vi "Process.vi"(8 "error in (no error)":errorcluster, 11 "SMO.UI":refnum<class "SMO.UI.lvclass">) -> (0 "error out":errorcluster, 3 "SMO.UI out":refnum<class "SMO.UI.lvclass">)   [LabVIEW 2019, in "SMO.UI.lvclass"]
doc: "JKI State Machine Objects (SMO) 1.3.0.56\nJKI - JKI\nCopyright (c) 2017, JKI"
uses:
  SMO.UI.lvclass
  C:/Users/Patrick/Documents/GitHub/Test (LV2019)/lv-venv/lv.lib/vi.lib/JKI/JKI SMO/SMO/SMO.lvclass
  SMO/Typedefs/Parent Call--Enum.ctl
  SMO/SMO.lvclass
  Typedefs/SMO.UI State--enum.ctl
panel:
  in  "self terminate":bool
  out "Copyright":string="JKI State Machine Objects™\nhttp://jki.net/state-machine-objects/\nCopyright (C) 2005-2015, JKI <info@jki.net>\nALL RIGHTS RESERVED\n\nFor instructions on how to use the JKI State Machine Objects, examples and video tutorials, visit:\nhttp://jki.net/state-machine-objects/\n"
  # "JKI SMO UI"
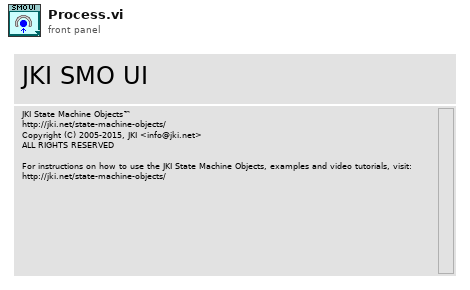
[diagram p1: front panel]
types:
  T1 = typedef "SMO.lvclass/Parent Call--Enum.ctl" = enum16{"Allows parent to run", "Does not request parent to run"}
  T2 = enum32{"invalid app kind", "Development System", "Run Time System", "Student Edition", "Embedded LabVIEW", "Evaluation", "Custom"}
  T3 = enum32{"Invalid", "Standard", "Closed", "Hidden", "Minimized", "Maximized"}
  T4 = typedef "SMO.UI.lvclass/SMO.UI State--enum.ctl" = enum16{"unknown", "Opened", "Closed"}
  T5 = cluster{"Core":cluster{"Current VI Reference":refnum<vi>, "Close Panel on Exit?":bool, "error":errorcluster}, "Self Ref":refnum<class "SMO.UI.lvclass">}
  T6 = cluster{"Current VI Reference":refnum<vi>, "Close Panel on Exit?":bool, "error":errorcluster}
  T7 = typedef "SMO.lvclass/Protected Events.ctl" = cluster{"StopProcesses":refnum<user-event>, "AbortProcesses":refnum<user-event>, "Config Changed":refnum<user-event>, "Dependency":refnum<user-event>}
  T8 = typedef "SMO.UI.lvclass/PrivateEvents--Cluster.ctl" = cluster{"Show-Hide UI":refnum<user-event>}
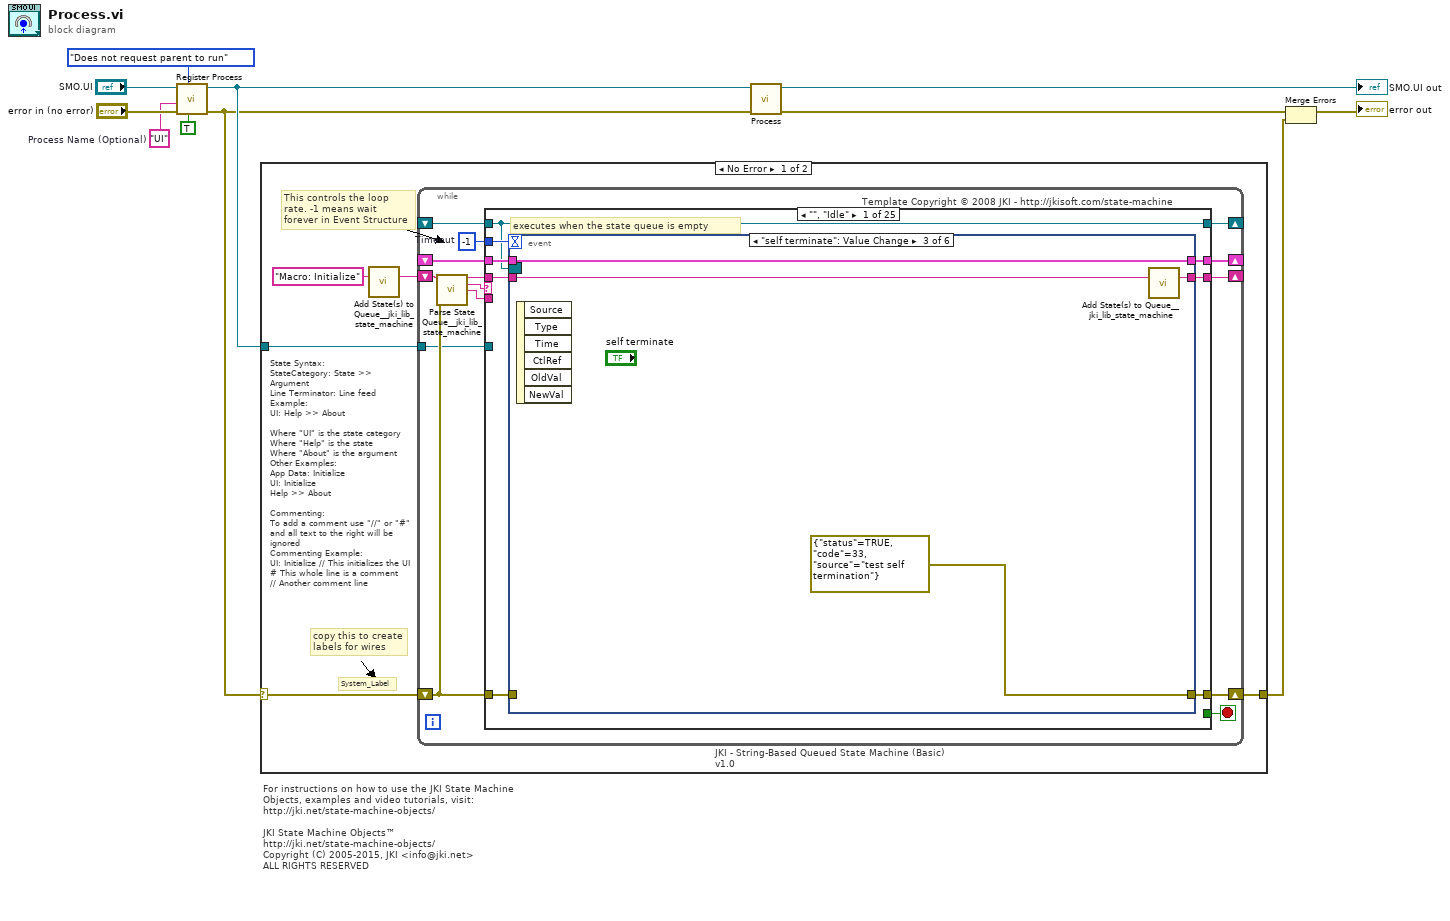
[diagram p0: block diagram]
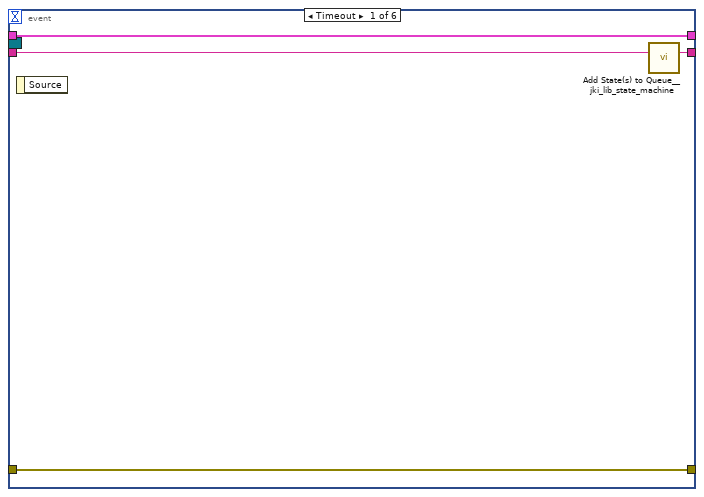
[diagram p2: hidden frame]
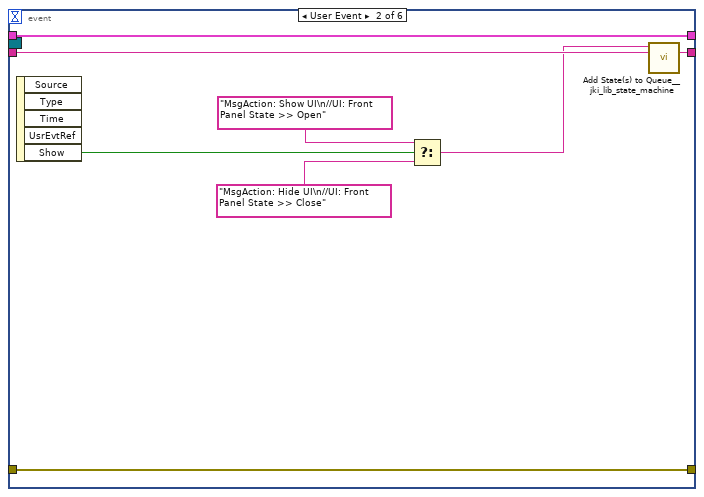
[diagram p3: hidden frame]
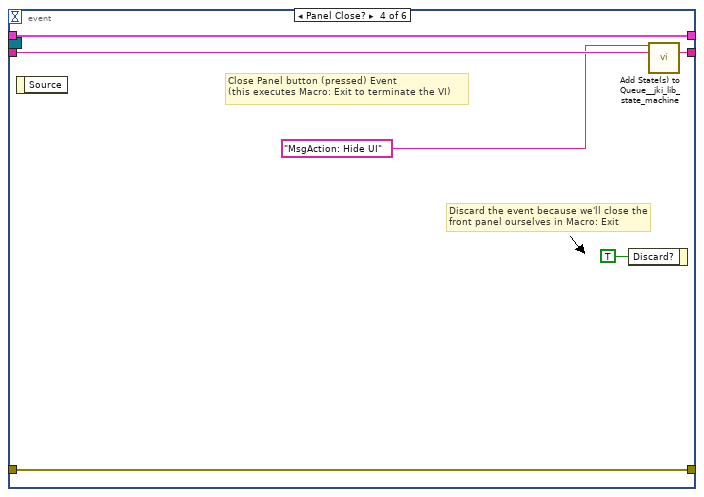
[diagram p4: hidden frame]
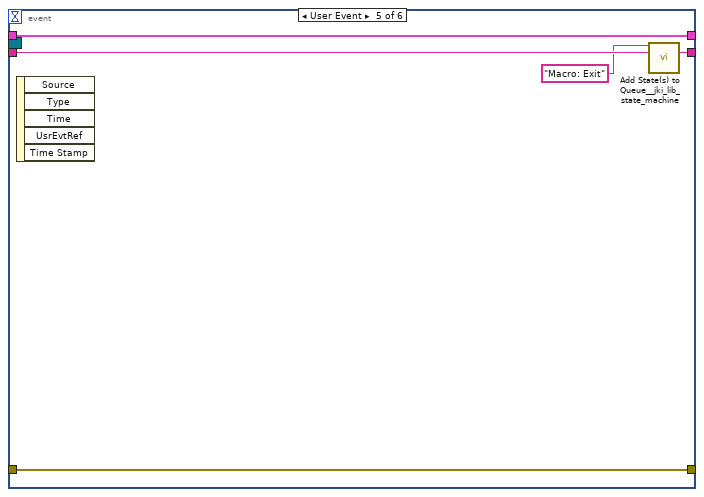
[diagram p5: hidden frame]
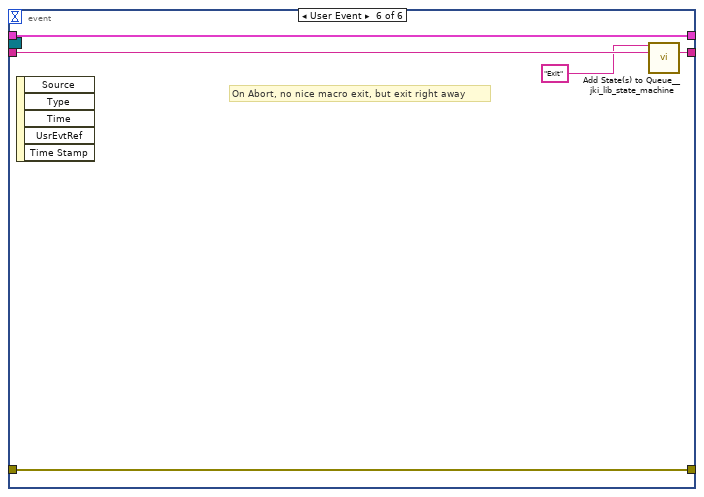
[diagram p6: hidden frame]
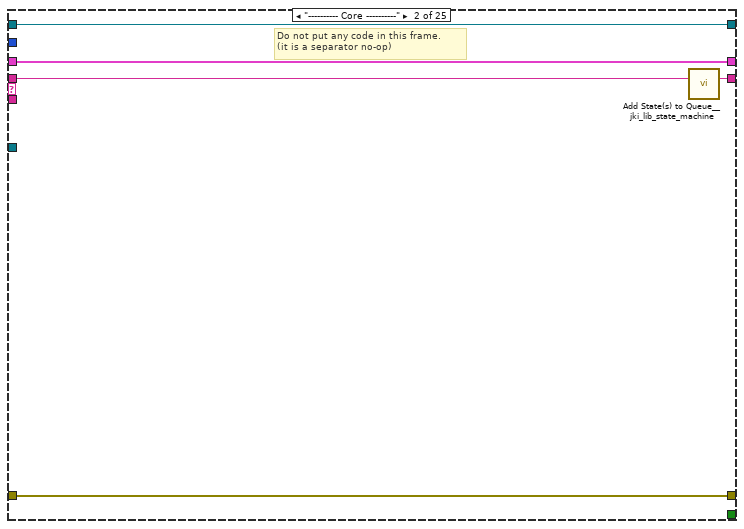
[diagram p7: hidden frame]
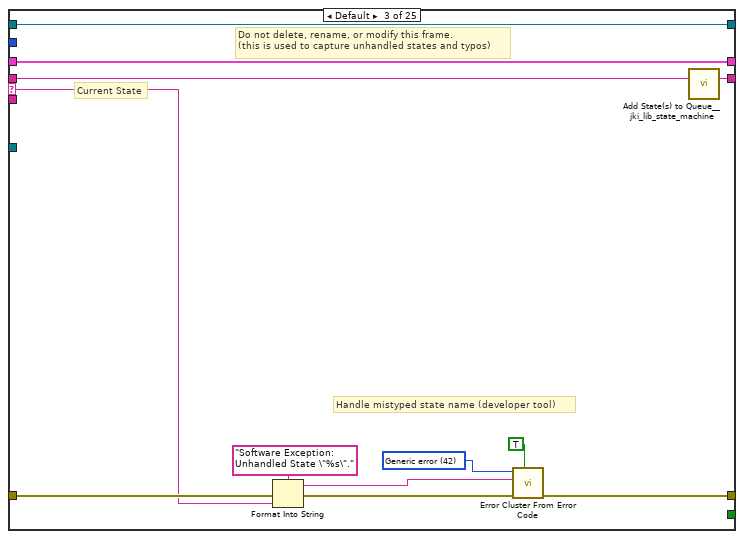
[diagram p8: hidden frame]
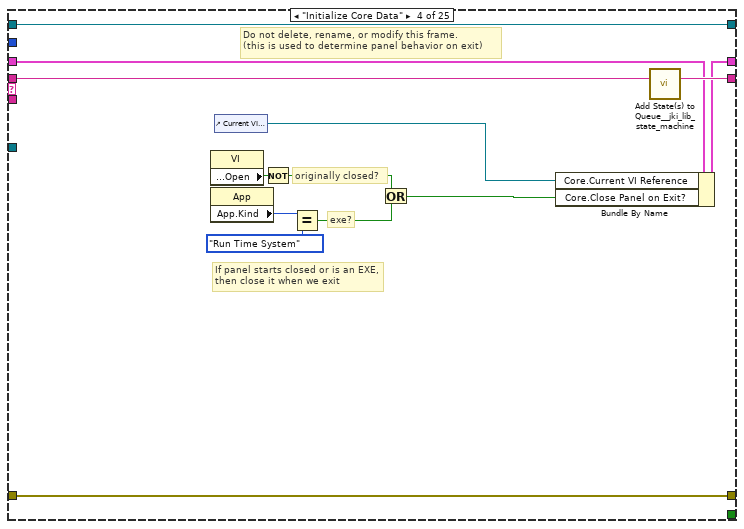
[diagram p9: hidden frame]
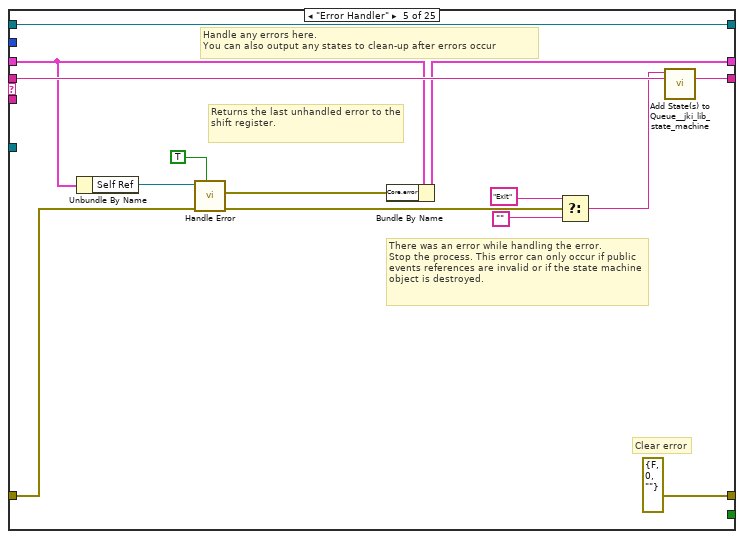
[diagram p10: hidden frame]
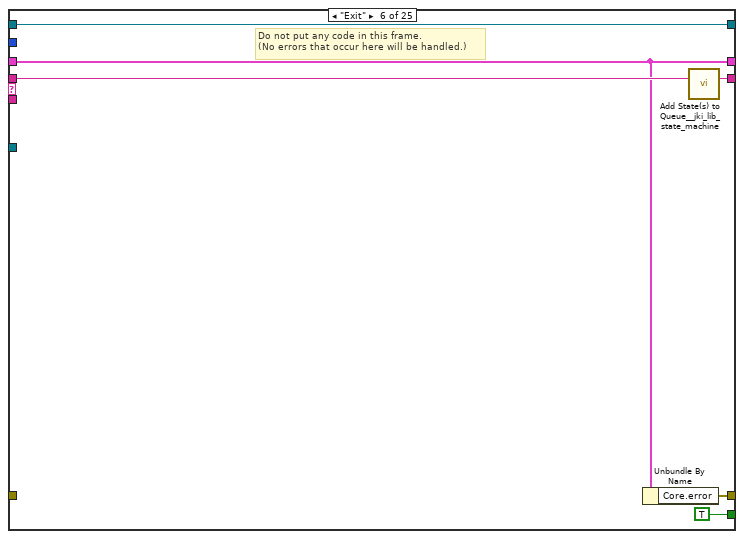
[diagram p11: hidden frame]
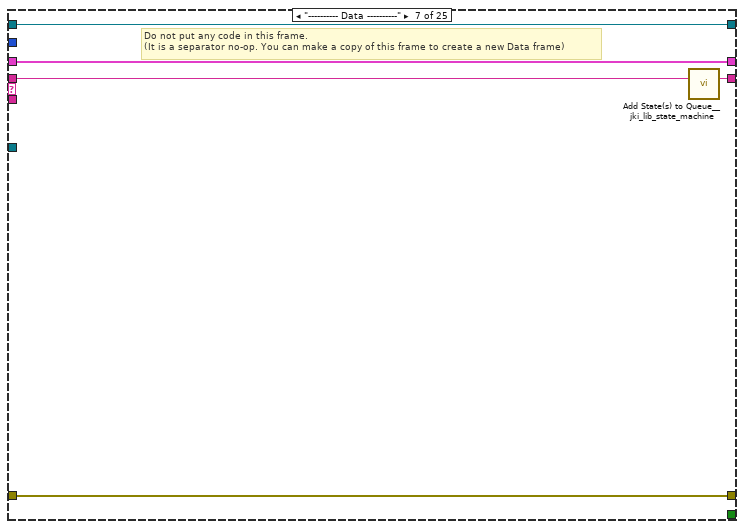
[diagram p12: hidden frame]
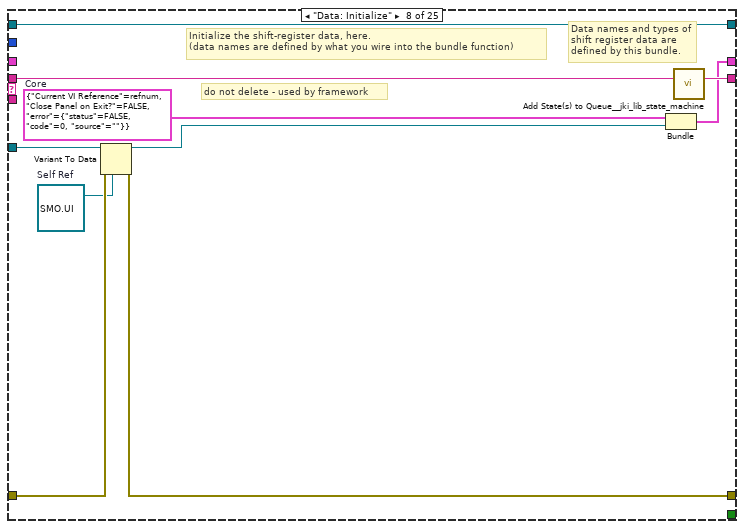
[diagram p13: hidden frame]
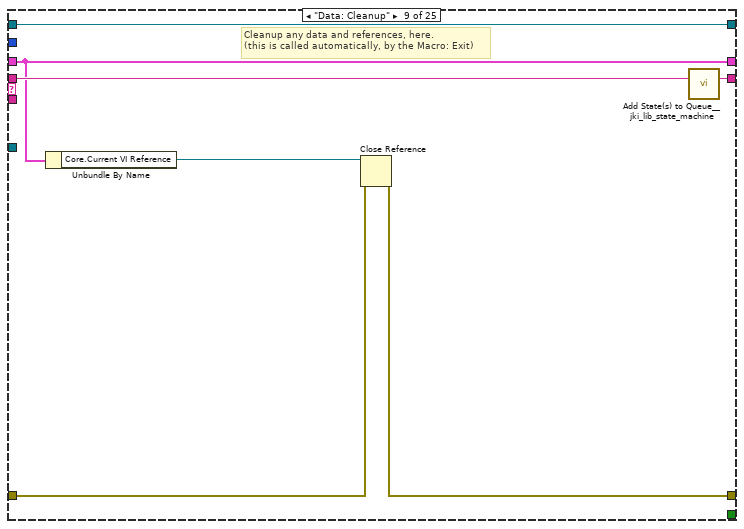
[diagram p14: hidden frame]
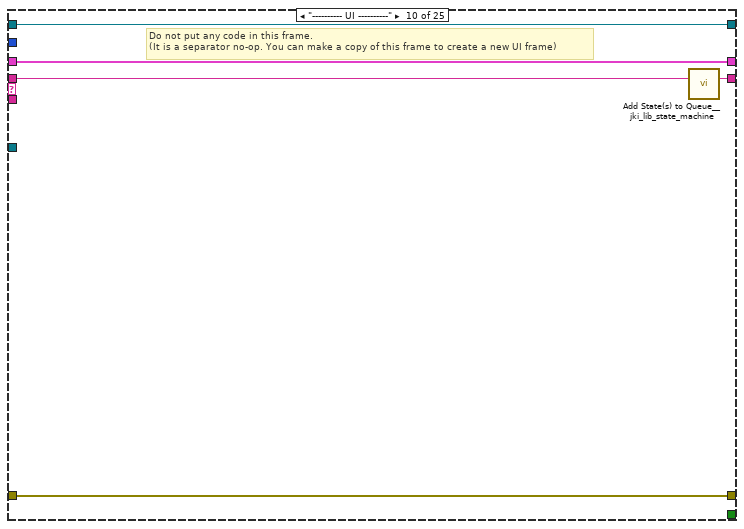
[diagram p15: hidden frame]
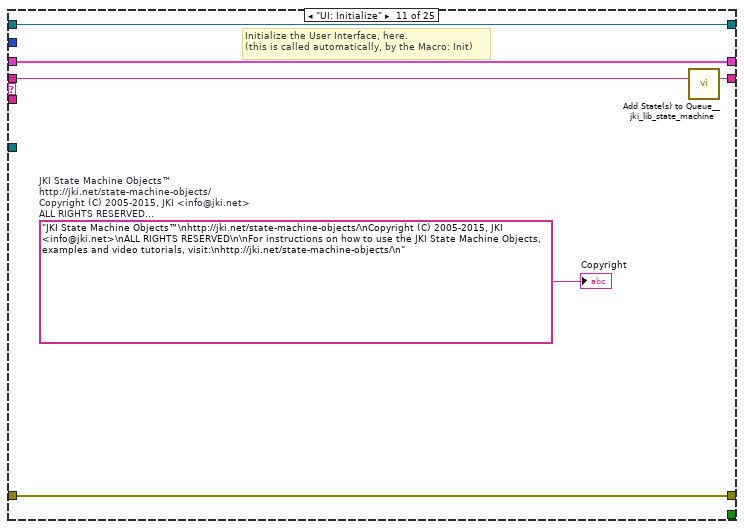
[diagram p16: hidden frame]
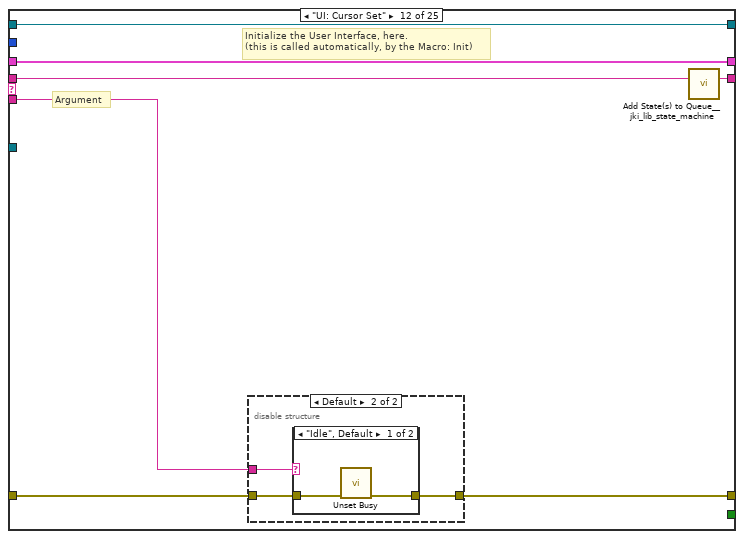
[diagram p17: hidden frame]
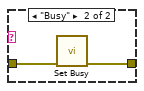
[diagram p19: hidden frame]
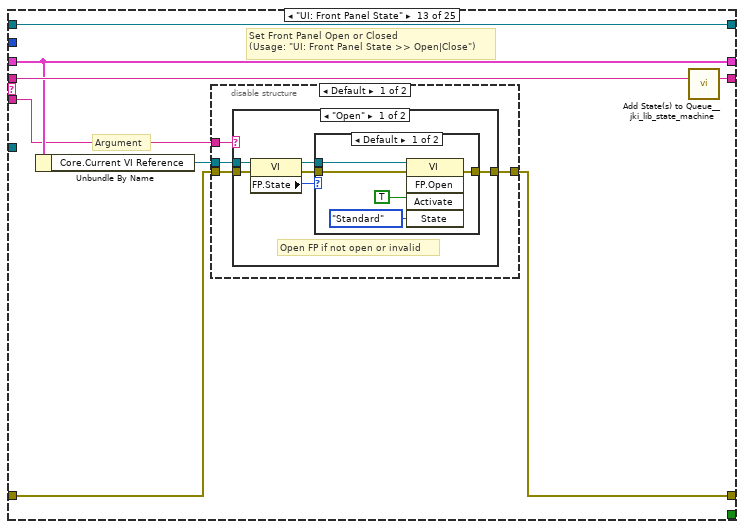
[diagram p20: hidden frame]
diagram:
  w4 = "UI"  # Process Name (Optional)
  # "For instructions on how to use the JKI State Machine Objects, examples and video tutorials, visit:\nhttp://jki.net/state-machine-objects/\n\nJKI State Machine Objects™\nhttp://jki.net/state-machine-objects/\nCopyright (C) 2005-2015, JKI <info@jki.net>\nALL RIGHTS RESERVED"
  n1 = call "Register Process.vi"("Forces Self to Run (F)"=TRUE, "Parent Call"=Parent_Call--Enum."Does not request parent to run", "error in (no error)"="error in (no error)", "Process Name (optional)"=w4, "SMO"="SMO.UI") -> ("error out"=w10:errorcluster, "SMO out"=w11:refnum<class "SMO.UI.lvclass">)  [unwired: 5 in]
  n2 = case shown="No Error" w10 {
    selector: w10 -> [w13 w317]
    tunnel: w11 -> [w14 _]
    tunnel: [w12 w317] -> w8
    frame No Error {
      # "State Syntax:\nStateCategory: State >> Argument\nLine Terminator: Line feed\nExample:\nUI: Help >> About\n\nWhere \"UI\" is the state category\nWhere \"Help\" is the state\nWhere \"About\" is the argument\nOther Examples:\nApp Data: Initialize\nUI: Initialize\nHelp >> About\n\nCommenting:\nTo add a comment use \"//\" or \"#\" and all text to the right will be ignored\nCommenting Example:\nUI: Initialize // This initializes the UI\n# This whole line is a comment\n// Another comment line"
      # "copy this to create labels for wires"
      # "This controls the loop rate. -1 means wait forever in Event Structure"
      # "System_Label"
      n3 = call "Add State(s) to Queue__jki_lib_state_machine.vi"("State(s) in (\"\")"="Macro: Initialize") -> ("States Out"=w16:string)  [unwired: 14 in]
      n4 = while "JKI - String-Based Queued State Machine (Basic) v1.0" {
        shift-right: [w23] -> _
        shift-left: _ -> [w22]
        shift-right: [w26] -> w12
        shift-left: w13 -> [w20]
        shift-right: [w25] -> _
        shift-left: w16 -> [w27]
        tunnel: w14 -> [w19]
        shift-right: [w18] -> _
        shift-left: _ -> [w17]
        stop <- w24 stop-if-true
        w21 = -1  # Timeout
        # "Template Copyright © 2008 JKI - http://jkisoft.com/state-machine"
        n5 = call "Parse State Queue__jki_lib_state_machine.vi"("State Queue"=w27, "Error In (no error)"=w20) -> ("Remaining States"=w29:string, "Current State"=w30:string, "Arguments"=w28:string)  [unwired: 11 in]
        n6 = case shown="\"\", \"Idle\"" w30 {
          selector: w30 -> [_ _ w77 _ _ _ _ _ _ _ _ _ _ _ _ _ _ _ _ _ _ _ _ _ _]
          tunnel: w29 -> [w38 w75 w81 w100 w114 w120 w125 w135 w142 w147 w153 w160 w176 w208 w217 w228 w233 w244 w256 w261 w273 w279 w284 w294 w309]
          tunnel: w28 -> [_ _ _ _ _ _ _ _ _ _ _ w154 w172 _ _ _ _ _ _ _ _ _ _ _ _]
          tunnel: w22 -> [w36 w72 w79 w91 w110 w115 w122 _ w137 w144 w151 w158 w174 w205 w213 w219 w230 w241 w253 w258 w271 w277 w281 w291 w306]
          tunnel: [w35 w73 w83 w97 errorcluster {"status"=FALSE, "code"=0, "source"=""} ("error out") w116 w123 w127 w138 w145 w150 w155 w169 w206 w215 w226 w231 w235 w251 w259 w269 w275 w282 w285 w300] -> w26
          tunnel: w20 -> [w34 w73 w82 w97 w107 _ w123 w132 w139 w145 w150 w156 w170 w206 w215 w226 w231 w236 w248 w259 w262 w275 w282 w289 w304]
          tunnel: [w37 w74 w80 w99 w113 w119 w124 w134 w141 w146 w152 w159 w175 w207 w216 w227 w232 w243 w255 w260 w272 w278 w283 w293 w308] -> w25
          tunnel: [_ _ _ _ _ TRUE _ _ _ _ _ _ _ _ _ _ _ _ _ _ _ _ _ _ _] -> w24
          tunnel: [w33 w72 w79 w98 w109 w115 w122 w133 w137 w144 w151 w158 w174 w205 w213 w219 w230 w241 w253 w258 w271 w277 w281 w291 w306] -> w23
          tunnel: w21 -> [w32 _ _ _ _ _ _ _ _ _ _ _ _ _ _ _ _ _ _ _ _ _ _ _ _]
          tunnel: w19 -> [_ _ _ _ _ _ _ w131 _ _ _ _ _ _ _ _ _ _ _ _ _ _ _ _ _]
          tunnel: [w31 w71 w76 w88 w112 w117 w121 w130 w136 w143 w149 w157 w173 w204 w214 w220 w229 w242 w254 w257 w268 w276 w280 w292 w307] -> w18
          tunnel: w17 -> [w31 w71 w76 w88 w112 w117 w121 w130 w136 w143 w149 w157 w173 w204 w214 w220 w229 w242 w254 w257 _ w276 w280 w292 w307]
          frame "", "Idle" {
            # "executes when the state queue is empty"
            n7 = event shown="[2] \"self terminate\": Value Change" {
              selector: w31 -> [_ _ _ _ _ _]
              dyn-events: _ -> [_ _ _ _ _ _]
              timeout: w32 -> [_ _ _ _ _ _]
              tunnel: w38 -> [w42 w50 w54 w60 w65 w70]
              tunnel: [w41 w49 w53 w59 w64 w69] -> w37
              tunnel: w36 -> [w39 w47 w52 w56 w62 w67]
              tunnel: [w40 w48 errorcluster {"status"=TRUE, "code"=33, "source"="test self termination"} ("error IO") w58 w63 w68] -> w35
              tunnel: w34 -> [w40 w48 _ w58 w63 w68]
              tunnel: [w39 w47 w52 w56 w62 w67] -> w33
              event Timeout {
                n8 = event-data() -> ()  [unwired: 1 in, 1 out]
                n9 = call "Add State(s) to Queue__jki_lib_state_machine.vi"("State(s) in (\"\")"=w42) -> ("States Out"=w41:string)  [unwired: 14 in]
              }
              event User Event {
                n10 = event-data() -> ("Show"=w46:bool)  [unwired: 1 in, 4 out]
                n11 = Select(t="MsgAction: Show UI\n//UI: Front Panel State >> Open" ("State(s) in Front (\"\")"), s=w46, f="MsgAction: Hide UI\n//UI: Front Panel State >> Close" ("State(s) in Front (\"\")")) -> (s? t:f=w43:string)
                n12 = call "Add State(s) to Queue__jki_lib_state_machine.vi"("State(s) in Front (\"\")"=w43, "State(s) in (\"\")"=w50) -> ("States Out"=w49:string)  [unwired: 13 in]
              }
              event "self terminate": Value Change {
                n13 = event-data() -> ()  [unwired: 1 in, 6 out]
                n14 = call "Add State(s) to Queue__jki_lib_state_machine.vi"("State(s) in (\"\")"=w54) -> ("States Out"=w53:string)  [unwired: 14 in]
              }
              event Panel Close? {
                # "Discard the event because we'll close the front panel ourselves in Macro: Exit"
                # "Close Panel button (pressed) Event\n(this executes Macro: Exit to terminate the VI)"
                n15 = event-data() -> ()  [unwired: 1 in, 1 out]
                n16 = event-data("Discard?"=TRUE) -> ()  [unwired: 1 in, 1 out]
                n17 = call "Add State(s) to Queue__jki_lib_state_machine.vi"("State(s) in Front (\"\")"="MsgAction: Hide UI", "State(s) in (\"\")"=w60) -> ("States Out"=w59:string)  [unwired: 13 in]
              }
              event User Event {
                n18 = event-data() -> ()  [unwired: 1 in, 5 out]
                n19 = call "Add State(s) to Queue__jki_lib_state_machine.vi"("State(s) in Front (\"\")"="Macro: Exit", "State(s) in (\"\")"=w65) -> ("States Out"=w64:string)  [unwired: 13 in]
              }
              event User Event {
                # "On Abort, no nice macro exit, but exit right away"
                n20 = event-data() -> ()  [unwired: 1 in, 5 out]
                n21 = call "Add State(s) to Queue__jki_lib_state_machine.vi"("State(s) in Front (\"\")"="Exit", "State(s) in (\"\")"=w70) -> ("States Out"=w69:string)  [unwired: 13 in]
              }
            }
          }
          frame "---------- Core ----------" {
            # "Do not put any code in this frame.\n(it is a separator no-op)"
            n22 = call "Add State(s) to Queue__jki_lib_state_machine.vi"("State(s) in (\"\")"=w75) -> ("States Out"=w74:string)  [unwired: 14 in]
          }
          frame Default {
            w86 = 42 items=["No error", "Argument error", "Memory is full", "Out of zone", "End of file", "File already open", "Generic file I/O error", "File not found", "File permission error", "Disk is full", "Duplicate path", "Too many files open", "System feature not enabled", "Resource file not found", "Cannot add resource", "Resource not found", "Image not found", "Image memory error", "Pen does not exist", "Config type invalid", "Config token not found", "Config parse error", "Config memory error", "Bad external code format", "Bad external code offset", "External code not present", "Null window", "Destroy window error", "Null menu", "Print aborted", "Bad print record", "Print driver error", "Windows error during printing", "Memory error during printing", "Print dialog error", "Generic print error", "Invalid device refnum", "Device not found", "Device parameter error", "Device unit error", "Cannot open device", "Device call aborted", "Generic error", "Cancelled by user", "Object ID too low", "Object ID too high", "Object not in heap", "Unknown heap", "Unknown object (invalid DefProc)", "Unknown object (DefProc not in table)", "Message out of range", "Invalid (null) method", "Unknown message", "Manager call not supported", "Bad address", "Network operation in progress", "Network operation timed out", "Connection is busy", "Network attribute not supported", "Network error", "Address in use", "System out of memory", "Connection aborted", "Connection refused", "Not connected", "Already connected", "Connection closed", "Initialization error (interapplication manager)", "Bad occurrence", "Wait on unbound occurrence handler", "Occurrence queue overflow", "Datalog type conflict", "Unused", "Unrecognized type (interapplication manager)", "Memory corrupt", "Failed to make temporary DLL", "Old CIN version", "Drag socket not found", "Failed to load drop-object", "Failed to register OLE object", "Failed to release OLE object", "Format specifier type mismatch", "Unknown format specifier", "Too few format specifiers", "Too many format specifiers", "Scan failed", "Newer CIN version", "Error converting to variant", "Runtime menu error", "Password tampered", "Variant attribute not found", "Incompatible variant data type", "Event data is not available", "Event Store is not present", "Occurrence is not found", "Event Queue is not created", "Event info is not available", "Refnum passed is NULL", "Error retrieving Class GUID", "Error retrieving CoClass GUID", "Error retrieving TypeLib GUID.", "Bad built application magic bytes.", "Specific driver is different from the specific driver associated with the Logical Name.", "There is no session opened to the class driver.", "Max Error", "MAX - Error with config objects", "MAX - Error loading configuration", "MAX - Group not supported"]
            # "Current State"
            # "Do not delete, rename, or modify this frame.\n(this is used to capture unhandled states and typos)"
            # "Handle mistyped state name (developer tool)"
            n23 = Format Into String(format string="Software Exception: Unhandled State \"%s\"." ("message"), error in=w82, w77) -> (resulting string=w85:string, error out=w84:errorcluster)  [unwired: 1 in]
            n24 = call <vilib>:"Error Cluster From Error Code.vi"("show call chain? (False)"=TRUE, "error in (no error)"=w84, "error message (\"\")"=w85, "error code (0)"=w86) -> ("error out"=w83:errorcluster)  [unwired: 5 in]
            n25 = call "Add State(s) to Queue__jki_lib_state_machine.vi"("State(s) in (\"\")"=w81) -> ("States Out"=w80:string)  [unwired: 14 in]
          }
          frame "Initialize Core Data" {
            # "Do not delete, rename, or modify this frame.\n(this is used to determine panel behavior on exit)"
            # "originally closed?"
            # "exe?"
            # "If panel starts closed or is an EXE, then close it when we exit"
            n26 = property class="VI"() -> ("Front Panel.Open"=w96:bool)  [unwired: 2 in, 2 out]
            n27 = property class="App"() -> ("App.Kind"=w95:T2)  [unwired: 2 in, 2 out]
            n28 = control-ref of="Current VI Reference"() -> (w89:refnum<vi>)
            n29 = Not(x=w96) -> (.not. x?=w93:bool)
            n30 = Equal?(x=w95, y=T2."Run Time System" ("Application:Kind")) -> (x = y?=w92:bool)
            n31 = Or(x=w93, y=w92) -> (x .or. y?=w90:bool)
            n32 = Bundle By Name(cluster=w91, "Core.Current VI Reference"=w89, "Core.Close Panel on Exit?"=w90) -> (w98:T5)
            n33 = call "Add State(s) to Queue__jki_lib_state_machine.vi"("State(s) in (\"\")"=w100) -> ("States Out"=w99:string)  [unwired: 14 in]
          }
          frame "Error Handler" {
            # "Returns the last unhandled error to the shift register."
            # "There was an error while handling the error.\nStop the process. This error can only occur if public events references are invalid or if the state machine object is destroyed."
            # "Handle any errors here.\nYou can also output any states to clean-up after errors occur"
            # "Clear error"
            n34 = Unbundle By Name(w110) -> ("Self Ref"=w111:refnum<class "SMO.UI.lvclass">)
            n35 = call-dynamic "Handle Error.vi"("Stop on Unhandled Error (T)"=TRUE, "error in"=w107, "SMO"=w111) -> ("handling error"=w105:errorcluster, "Unhandled error"=w108:errorcluster)  [unwired: 6 in, 1 out]
            n36 = Bundle By Name(cluster=w110, "Core.error"=w108) -> (w109:T5)
            n37 = Select(t="Exit", s=w105, f="") -> (s? t:f=w102:string)
            n38 = call "Add State(s) to Queue__jki_lib_state_machine.vi"("State(s) in Front (\"\")"=w102, "State(s) in (\"\")"=w114) -> ("States Out"=w113:string)  [unwired: 13 in]
          }
          frame "Exit" {
            # "Do not put any code in this frame.\n(No errors that occur here will be handled.)"
            n39 = Unbundle By Name(w115) -> ("Core.error"=w116:errorcluster)
            n40 = call "Add State(s) to Queue__jki_lib_state_machine.vi"("State(s) in (\"\")"=w120) -> ("States Out"=w119:string)  [unwired: 14 in]
          }
          frame "---------- Data ----------" {
            # "Do not put any code in this frame.\n(It is a separator no-op. You can make a copy of this frame to create a new Data frame)"
            n41 = call "Add State(s) to Queue__jki_lib_state_machine.vi"("State(s) in (\"\")"=w125) -> ("States Out"=w124:string)  [unwired: 14 in]
          }
          frame "Data: Initialize" {
            w126 = T6 {"Current VI Reference"=refnum, "Close Panel on Exit?"=FALSE, "error"={"status"=FALSE, "code"=0, "source"=""}}  # Core
            w129 = refnum<class "SMO.UI.lvclass"> refnum  # Self Ref
            # "do not delete - used by framework"
            # "Data names and types of shift register data are defined by this bundle."
            # "Initialize the shift-register data, here.\n(data names are defined by what you wire into the bundle function)"
            n42 = Variant To Data(error in=w132, type=w129, Variant=w131) -> (data=w128:refnum<class "SMO.UI.lvclass">, error out=w127:errorcluster)
            n43 = Bundle("Core"=w126, "Self Ref"=w128) -> (w133:T5)  [unwired: 1 in]
            n44 = call "Add State(s) to Queue__jki_lib_state_machine.vi"("State(s) in (\"\")"=w135) -> ("States Out"=w134:string)  [unwired: 14 in]
          }
          frame "Data: Cleanup" {
            # "Cleanup any data and references, here.\n(this is called automatically, by the Macro: Exit)"
            n45 = Unbundle By Name(w137) -> ("Core.Current VI Reference"=w140:refnum<vi>)
            n46 = Close Reference(reference=w140, error in (no error)=w139) -> (error out=w138:errorcluster)
            n47 = call "Add State(s) to Queue__jki_lib_state_machine.vi"("State(s) in (\"\")"=w142) -> ("States Out"=w141:string)  [unwired: 14 in]
          }
          frame "---------- UI ----------" {
            # "Do not put any code in this frame.\n(It is a separator no-op. You can make a copy of this frame to create a new UI frame)"
            n48 = call "Add State(s) to Queue__jki_lib_state_machine.vi"("State(s) in (\"\")"=w147) -> ("States Out"=w146:string)  [unwired: 14 in]
          }
          frame "UI: Initialize" {
            w148 = "JKI State Machine Objects™\nhttp://jki.net/state-machine-objects/\nCopyright (C) 2005-2015, JKI <info@jki.net>\nALL RIGHTS RESERVED\n\nFor instructions on how to use the JKI State Machine Objects, examples and video tutorials, visit:\nhttp://jki.net/state-machine-objects/\n"  # JKI State Machine Objects™ http://jki.net/state-machine-objects/ Copyright (C) 2005-2015, JKI <info@jki.net> ALL RIGHTS RESERVED  For instructions on how to use the JKI State Machine Objects, examples and video tutorials, visit: http://jki.net/state-machine-objects/
            # "Initialize the User Interface, here.\n(this is called automatically, by the Macro: Init)"
            n49 = call "Add State(s) to Queue__jki_lib_state_machine.vi"("State(s) in (\"\")"=w153) -> ("States Out"=w152:string)  [unwired: 14 in]
            "Copyright" <- w148
          }
          frame "UI: Cursor Set" {
            # "Argument"
            # "Initialize the User Interface, here.\n(this is called automatically, by the Macro: Init)"
            n50 = disable-structure shown="Default" {
              disable-tunnel: w156 -> [w161 w164]
              disable-tunnel: [w161 w163] -> w155
              disable-tunnel: w154 -> [_ w162]
              frame condition #0 {
              }
              frame condition #1 (active) {
                n51 = case shown="\"Idle\", Default" w162 {
                  tunnel: w164 -> [w166 w168]
                  tunnel: [w165 w167] -> w163
                  frame "Idle", Default {
                    n52 = call <vilib>:"Unset Busy.vi"("error in (no error)"=w166) -> ("error out"=w165:errorcluster)  [unwired: 10 in]
                  }
                  frame "Busy" {
                    n53 = call <vilib>:"Set Busy.vi"("error in (no error)"=w168) -> ("error out"=w167:errorcluster)  [unwired: 9 in, 1 out]
                  }
                }
              }
            }
            n54 = call "Add State(s) to Queue__jki_lib_state_machine.vi"("State(s) in (\"\")"=w160) -> ("States Out"=w159:string)  [unwired: 14 in]
          }
          frame "UI: Front Panel State" {
            # "Argument"
            # "Set Front Panel Open or Closed\n(Usage: \"UI: Front Panel State >> Open|Close\")"
            n55 = Unbundle By Name(w174) -> ("Core.Current VI Reference"=w171:refnum<vi>)
            n56 = disable-structure shown="Default" {
              disable-tunnel: w170 -> [w180 w203]
              disable-tunnel: [w179 w203] -> w169
              disable-tunnel: w171 -> [w178 _]
              disable-tunnel: w172 -> [w177 _]
              frame condition #0 (active) {
                n57 = case shown="\"Open\"" w177 {
                  tunnel: w180 -> [w184 w197]
                  tunnel: [w186 w198] -> w179
                  tunnel: w178 -> [w185 w195]
                  frame "Open" {
                    # "Open FP if not open or invalid"
                    n58 = property class="VI"(reference=w185, error in=w184) -> (reference out=w182:refnum<vi>, error out=w183:errorcluster, "FP.State"=w181:T3)
                    n59 = case shown="Default" w181 {
                      tunnel: [w189 w192] -> w186
                      tunnel: w183 -> [w188 w192]
                      tunnel: w182 -> [w187 _]
                      frame Default {
                        n60 = invoke class="VI" method="FP.Open"(reference=w187, error in=w188, "Activate"=TRUE, "State"=T3."Standard") -> (error out=w189:errorcluster)  [unwired: 1 in, 4 out]
                      }
                      frame "Invalid", "Standard" {
                      }
                    }
                  }
                  frame "Close", Default {
                    # "Close FP is not Closed or Invalid"
                    n61 = property class="VI"(reference=w195, error in=w197) -> (reference out=w194:refnum<vi>, error out=w196:errorcluster, "FP.State"=w193:T3)
                    n62 = case shown="Default" w193 {
                      tunnel: [w199 w202] -> w198
                      tunnel: w196 -> [w199 w201]
                      tunnel: w194 -> [_ w200]
                      frame "Invalid", "Closed" {
                      }
                      frame Default {
                        n63 = invoke class="VI" method="FP.Close"(reference=w200, error in=w201) -> (error out=w202:errorcluster)  [unwired: 1 in, 2 out]
                      }
                    }
                  }
                }
              }
              frame condition #1 {
              }
            }
            n64 = call "Add State(s) to Queue__jki_lib_state_machine.vi"("State(s) in (\"\")"=w176) -> ("States Out"=w175:string)  [unwired: 14 in]
          }
          frame "---------- Macro ----------" {
            # "Do not put any code in this frame.\n(It is a separator no-op. You can make a copy of this frame to create a new Macro frame)"
            n65 = call "Add State(s) to Queue__jki_lib_state_machine.vi"("State(s) in (\"\")"=w208) -> ("States Out"=w207:string)  [unwired: 14 in]
          }
          frame "Macro: Initialize" {
            w211 = "UI: Initialize\n//UI: Front Panel State >> Open\n\n//Test: Start SMO Dependency //Only for development purpose."  # UI: Initialize //UI: Front Panel State >> Open  //Test: Start SMO Dependency //Only for development purpose.
            # "Initialization Macro\n(This is called once, when the VI starts)"
            n66 = call "Add State(s) to Queue__jki_lib_state_machine.vi"("State(s) in Front (\"\")"="Data: Initialize\nInitialize Core Data\nEvents: Register", "State(s) in (\"\")"="Process: Sync", "State(s) at Back (\"\")"=w211) -> ("States Out"=w210:string)  [unwired: 12 in]
            n67 = call "Add State(s) to Queue__jki_lib_state_machine.vi"("State(s) in Front (\"\")"=w210, "State(s) in (\"\")"=w217) -> ("States Out"=w216:string)  [unwired: 13 in]
          }
          frame "Macro: Exit" {
            # "Exit Macro\n(This is called once, when the VI exits)"
            n68 = Unbundle By Name(w219) -> ("Core.Close Panel on Exit?"=w225:bool)
            n69 = Select(t="UI: Front Panel State >> Close", s=w225, f="") -> (s? t:f=w222:string)
            n70 = call "Add State(s) to Queue__jki_lib_state_machine.vi"("State(s) in (\"\")"=w222, "State(s) at Back (\"\")"="Data: Cleanup\nEvents: Unregister\nProcess: Sync\nExit") -> ("States Out"=w221:string)  [unwired: 13 in]
            n71 = call "Add State(s) to Queue__jki_lib_state_machine.vi"("State(s) in Front (\"\")"=w221, "State(s) in (\"\")"=w228) -> ("States Out"=w227:string)  [unwired: 13 in]
          }
          frame "---------- Process ----------" {
            # "Template Separator\n(You can make a copy of, or modify, this frame)"
            n72 = call "Add State(s) to Queue__jki_lib_state_machine.vi"("State(s) in (\"\")"=w233) -> ("States Out"=w232:string)  [unwired: 14 in]
          }
          frame "Process: Sync" {
            n73 = Unbundle By Name(w241) -> ("Self Ref"=w237:refnum<class "SMO.UI.lvclass">)
            n74 = call "WaitOnProcessSync.vi"("error in (no error)"=w236, "SMO"=w237) -> ("error out"=w235:errorcluster, "Don't run?"=w240:bool)  [unwired: 7 in, 1 out]
            n75 = Select(t="Data: Cleanup\nEvents: Unregister\nExit", s=w240, f="") -> (s? t:f=w234:string)
            n76 = call "Add State(s) to Queue__jki_lib_state_machine.vi"("State(s) in Front (\"\")"=w234, "State(s) in (\"\")"=w244) -> ("States Out"=w243:string)  [unwired: 13 in]
          }
          frame "Test: Start SMO Dependency" {
            # ">> Returns the instance of \"Dummy\"\nand ignores the other levels dependencies"
            n77 = Unbundle By Name(w253) -> ("Self Ref"=w252:refnum<class "SMO.UI.lvclass">)
            n78 = call "LaunchDependency.vi"("error in (no error)"=w248, "Dependency Name"="Dummy", "Dependency Type"=refnum<class "SMO.lvclass"> refnum ("SMO.lvclass"), "SMO in"=w252) -> ("error out"=w251:errorcluster, "SMO out"=w245:refnum<class "SMO.UI.lvclass">)  [unwired: 4 in, 2 out]
            n79 = call "ListThisLevelDependencies.vi"("SMO in"=w245) -> ("[My Dependencies]"=w247:refnum<class "SMO.lvclass">[])  [unwired: 8 in, 2 out]
            n80 = Index Array(array=w247) -> (element=w246:refnum<class "SMO.lvclass">)  [unwired: 1 in]
            n81 = call "Get Name.vi"("SMO"=w246) -> ()  [unwired: 8 in, 3 out]
            n82 = call "Add State(s) to Queue__jki_lib_state_machine.vi"("State(s) in (\"\")"=w256) -> ("States Out"=w255:string)  [unwired: 14 in]
          }
          frame "---------- Events ----------" {
            # "Template Separator\n(You can make a copy of, or modify, this frame)"
            n83 = call "Add State(s) to Queue__jki_lib_state_machine.vi"("State(s) in (\"\")"=w261) -> ("States Out"=w260:string)  [unwired: 14 in]
          }
          frame "Events: Register" {
            n84 = Unbundle By Name(w271) -> ("Self Ref"=w267:refnum<class "SMO.UI.lvclass">)
            n85 = call "GetProtectedEvents.vi"("error in (no error)"=w262, "SMO"=w267) -> ("error out"=w263:errorcluster, "SMO Protected Events"=w270:T7, "SMO out"=w264:refnum<class "SMO.UI.lvclass">)  [unwired: 7 in]
            n86 = call "SMO.UI.GetPrivateEvents.vi"("error in (no error)"=w263, "SMO.UI"=w264) -> ("error out"=w265:errorcluster, "SMO.UI Private Events"=w266:T8)  [unwired: 7 in, 1 out]
            n87 = register-events(error in=w265, w270, w266) -> (reference out=w268:refnum<event-registration>, error out=w269:errorcluster)  [unwired: 1 in]
            n88 = call "Add State(s) to Queue__jki_lib_state_machine.vi"("State(s) in (\"\")"=w273) -> ("States Out"=w272:string)  [unwired: 14 in]
          }
          frame "Events: Unregister" {
            # "Your code here.\n(You can make a copy of, or modify, this frame)"
            n89 = Unregister For Events(event registration refnum=w276, error in=w275) -> (error out=w274:errorcluster)
            n90 = call <vilib>:"Clear Errors.vi"("error in (no error)"=w274) -> ()  [unwired: 5 in, 2 out]
            n91 = call "Add State(s) to Queue__jki_lib_state_machine.vi"("State(s) in (\"\")"=w279) -> ("States Out"=w278:string)  [unwired: 14 in]
          }
          frame "---------MsgAction---------" {
            # "MsgAction Separator\n(You can make a copy of, or modify, this frame)"
            n92 = call "Add State(s) to Queue__jki_lib_state_machine.vi"("State(s) in (\"\")"=w284) -> ("States Out"=w283:string)  [unwired: 14 in]
          }
          frame "MsgAction: Show UI" {
            n93 = Unbundle By Name(w291) -> ("Self Ref"=w290:refnum<class "SMO.UI.lvclass">)
            n94 = call-dynamic "Show User Interface.vi"("error in (no error)"=w289, "Show UI"=TRUE, "SMO.UI"=w290) -> ("error out"=w286:errorcluster, "SMO.UI out"=w287:refnum<class "SMO.UI.lvclass">)  [unwired: 7 in]
            n95 = case shown="No Error" w286 {
              selector: w286 -> [w297 w299]
              tunnel: w287 -> [w298 _]
              tunnel: [w296 w299] -> w285
              frame No Error {
                n96 = call "NotifyUIState.vi"("error in (no error)"=w297, "UI State"=SMO.UI_State--enum."Opened", "SMO.UI"=w298) -> ("error out"=w296:errorcluster)  [unwired: 7 in, 1 out]
              }
              frame Error {
              }
            }
            n97 = call "Add State(s) to Queue__jki_lib_state_machine.vi"("State(s) in (\"\")"=w294) -> ("States Out"=w293:string)  [unwired: 14 in]
          }
          frame "MsgAction: Hide UI" {
            n98 = Unbundle By Name(w306) -> ("Self Ref"=w305:refnum<class "SMO.UI.lvclass">)
            n99 = call-dynamic "Show User Interface.vi"("error in (no error)"=w304, "Show UI"=FALSE, "SMO.UI"=w305) -> ("error out"=w301:errorcluster, "SMO.UI out"=w302:refnum<class "SMO.UI.lvclass">)  [unwired: 7 in]
            n100 = case shown="No Error" w301 {
              selector: w301 -> [w314 w316]
              tunnel: w302 -> [w315 _]
              tunnel: [w310 w316] -> w300
              frame No Error {
                n101 = call "NotifyUIHidden.vi"("error in (no error)"=w314, "SMO.UI"=w315) -> ("error out"=w311:errorcluster, "SMO.UI out"=w312:refnum<class "SMO.UI.lvclass">)  [unwired: 8 in]
                n102 = call "NotifyUIState.vi"("error in (no error)"=w311, "UI State"=SMO.UI_State--enum."Closed", "SMO.UI"=w312) -> ("error out"=w310:errorcluster)  [unwired: 7 in, 1 out]
              }
              frame Error {
              }
            }
            n103 = call "Add State(s) to Queue__jki_lib_state_machine.vi"("State(s) in (\"\")"=w309) -> ("States Out"=w308:string)  [unwired: 14 in]
          }
        }
      }
    }
    frame Error {
    }
  }
  n104 = call-parent "Process.vi"("error in"=w10, "SMO"=w11) -> ("error out"=w9:errorcluster, "SMO out"=→"SMO.UI out":refnum<class "SMO.UI.lvclass">)  [unwired: 8 in]
  n105 = Merge Errors(w9, w8) -> (→"error out":errorcluster)
